vi "FTW-JSON-Object-Keys.vi"(0 "JSON Object":refnum<data-value>, 11 "error in":errorcluster) -> (4 "JSON Object out":refnum<data-value>, 6 "Keys":string[](array[string]), 8 "Elements":i64[](array[numeric]) format="%016x", 15 "error out":errorcluster)   [LabVIEW 2014]
uses:
  core/FTW-JSON-Core-Structure.ctl
  error/FTW-ERR-ThrowGenericError.vi
  error/FTW-ERR-ThrowError.vi
  error/FTW-ERR-NoErrorConstant.vi
  error/FTW-ERR-CallChain.vi
  string/FTW-STR-ReplaceWhitespace.vi
panel:
  # "Inputs"
  # "Outputs"
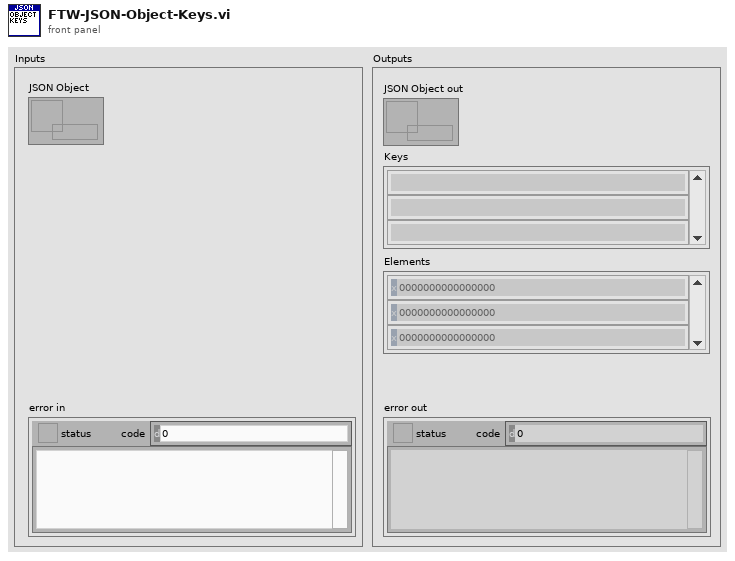
[diagram p1: front panel]
types:
  T1 = typedef "FTW-JSON-Core-Structure.ctl" = cluster{"JSON Object":i64, "Encoding Flags":i64, "Decoding Flags":i64}
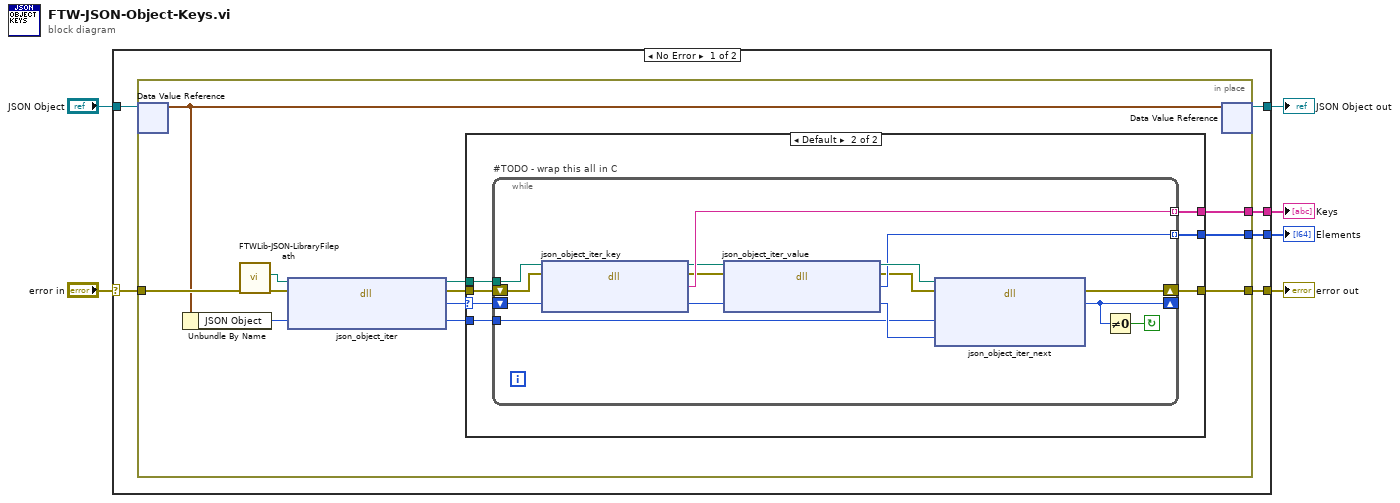
[diagram p0: block diagram]
diagram:
  n1 = case shown="No Error" "error in" {
    selector: "error in" -> [w9 w49]
    tunnel: [w12 w49] -> w6
    tunnel: [w7 w48] -> w4
    tunnel: "JSON Object" -> [w8 w48]
    tunnel: [w11 _] -> w2
    tunnel: [w10 _] -> w1
    frame No Error {
      n2 = in-place {
        in-place-border: [w24] -> w12
        in-place-border: [w23] -> w11
        in-place-border: [w22] -> w10
        in-place-border: w9 -> [w20]
        n3 = in-place-dvr #1(w8) -> (w13:T1)  [unwired: 1 out]
        n4 = Unbundle By Name(w13) -> ("JSON Object"=w17:i64)
        n5 = call "FTWLib-JSON-LibraryFilepath.vi"("error in"=w20) -> ("error out"=w19:errorcluster, "JSON Library Filepath"=w18:path)  [unwired: 9 in]
        n6 = dll-call lib="?" fn="json_object_iter"(path in=w18, error in=w19, "JSON Object Pointer"=w17) -> (path out=w15:path, error out=w21:errorcluster, "JSON Object Iterator Pointer"=w14:i64, "JSON Object Pointer"=w16:i64)  [unwired: 1 in]
        n7 = case shown="Default" w14 {
          selector: w14 -> [_ w26]
          tunnel: [w25 w32] -> w24
          tunnel: [_ w31] -> w23
          tunnel: [_ w30] -> w22
          tunnel: w21 -> [w25 w29]
          tunnel: w16 -> [_ w28]
          tunnel: w15 -> [_ w27]
          frame 0 {
          }
          frame Default {
            n8 = while "#TODO - wrap this all in C" {
              tunnel: [w46] -> w30 mode=indexing
              tunnel: [w35] -> w31 mode=indexing
              shift-right: [w47] -> w32
              shift-left: w29 -> [w38]
              tunnel: w28 -> [w40]
              tunnel: w27 -> [w39]
              shift-right: [w36] -> _
              shift-left: w26 -> [w37]
              stop <- w33 continue-if-true
              n9 = dll-call lib="?" fn="json_object_iter_key"(path in=w39, error in=w38, "JSON Iterator Pointer"=w37) -> (path out=w44:path, error out=w43:errorcluster, "Current Key"=w46:string, "JSON Iterator Pointer"=w42:i64)  [unwired: 1 in]
              n10 = dll-call lib="?" fn="json_object_iter_value"(path in=w44, error in=w43, "JSON Iterator Pointer"=w42) -> (path out=w41:path, error out=w34:errorcluster, "JSON Object Pointer"=w35:i64, "JSON Iterator Pointer"=w45:i64)  [unwired: 1 in]
              n11 = dll-call lib="?" fn="json_object_iter_next"(path in=w41, error in=w34, "JSON Object Pointer"=w40, "JSON Iterator Pointer"=w45) -> (error out=w47:errorcluster, "Next JSON Iterator Pointer"=w36:i64)  [unwired: 3 in, 1 out]
              n12 = Not Equal To 0?(x=w36) -> (x != 0?=w33:bool)
            }
          }
        }
        n13 = in-place-dvr #1(w13) -> (w7:refnum<data-value>)  [unwired: 1 out]
      }
    }
    frame Error {
    }
  }
  "error out" <- w6
  "JSON Object out" <- w4
  "Elements" <- w2
  "Keys" <- w1
